vi "Get Pos Impl.vi"(8 "error in (no error)":errorcluster, 11 "ASI Stage in":refnum<class "ASI Stage.lvclass">) -> (0 "error out":errorcluster, 2 "Stage Position":T1, 3 "ASI Stage out":refnum<class "ASI Stage.lvclass">)   [LabVIEW 2023, in "ASI Stage.lvlib" / "ASI Stage.lvclass"]
uses:
  ASI Stage.lvclass
  Resources/Type Defs/Stage Position.ctl
  <instrlib>/ASI TG-1000/ASI TG-1000.lvlib
  <instrlib>/ASI TG-1000/Public/Utility/Axis Name.ctl
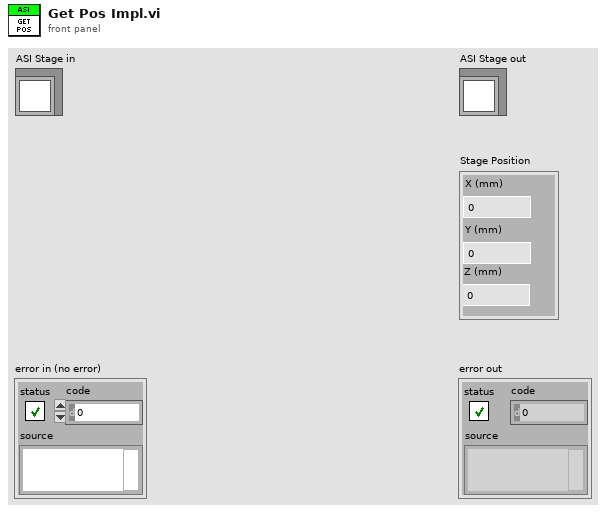
[diagram p1: front panel]
types:
  T1 = typedef "Stage Position.ctl" = cluster{"X (mm)":dbl, "Y (mm)":dbl, "Z (mm)":dbl}
  T2 = typedef "ASI TG-1000.lvlib/Axis Name.ctl" = enum8{"undefined", "A", "B", "C", "D", "E", "F", "G", "H", "I", "J", "K", "L", "M", "N", "O", "P", "Q", "R", "S", "T", "U", "V", "W", "X", "Y", "Z"}
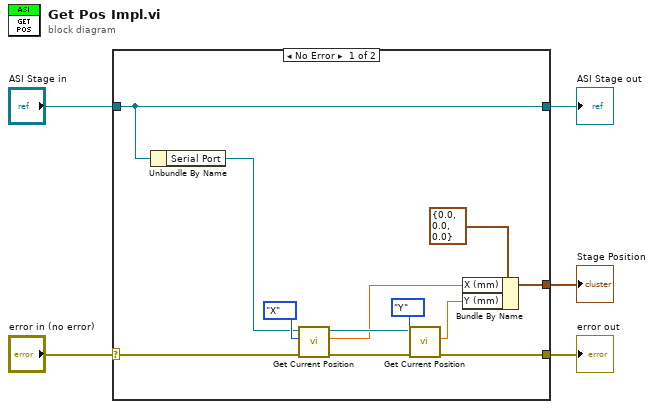
[diagram p0: block diagram]
diagram:
  n1 = case shown="No Error" "error in (no error)" {
    selector: "error in (no error)" -> [w11 w18]
    tunnel: [w8 w18] -> w4
    tunnel: "ASI Stage in" -> [w10 w19]
    tunnel: [w10 w19] -> w2
    tunnel: [w17 _] -> w1
    frame No Error {
      n2 = Unbundle By Name(w10) -> ("Serial Port"=w9:refnum<visa-resource-name>)
      n3 = call <instrlib>:"Get Current Position.vi"("error in (no error)"=w11, "Axis"=Axis_Name."X", "VISA in"=w9) -> ("error out"=w15:errorcluster, "position [internal units]"=w6:dbl, "VISA out"=w12:refnum<visa-resource-name>)  [unwired: 6 in]
      n4 = call <instrlib>:"Get Current Position.vi"("error in (no error)"=w15, "Axis"=Axis_Name."Y", "VISA in"=w12) -> ("error out"=w8:errorcluster, "position [internal units]"=w7:dbl)  [unwired: 6 in, 1 out]
      n5 = Bundle By Name(cluster=T1 {"X (mm)"=0.0, "Y (mm)"=0.0, "Z (mm)"=0.0} ("Stage Position 2"), "X (mm)"=w6, "Y (mm)"=w7) -> (w17:T1)
    }
    frame Error {
    }
  }
  "error out" <- w4
  "ASI Stage out" <- w2
  "Stage Position" <- w1
